vi "newRampTime.vi"(8 "error in (no error)":errorcluster, 11 "RampAction in":refnum<class "RampAction.lvclass">) -> (0 "error out":errorcluster, 3 "RampAction out":refnum<class "RampAction.lvclass">)   [LabVIEW 2009, in "Views.lvlib" / "ScriptEditor.lvlib" / "RampAction.lvclass"]
uses:
  RampAction.lvclass
  RampAction.lvclass/RampAction.ctl
  Tools/Scripting/ScriptingEvent/ScriptEvents/Ramp/RampEvent/RampEvent.lvclass
  ActionPanel.lvclass
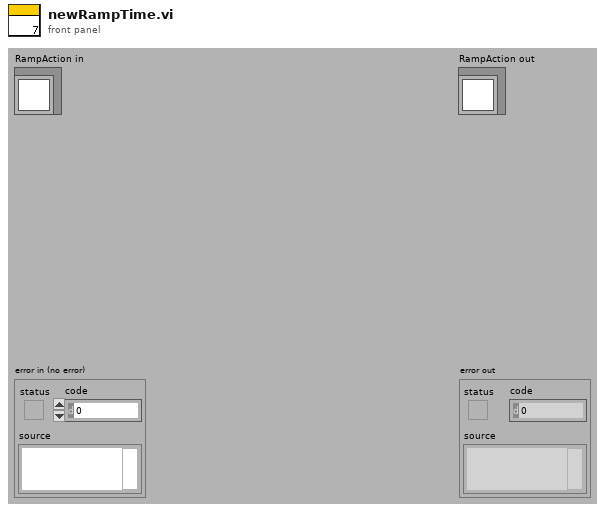
[diagram p1: front panel]
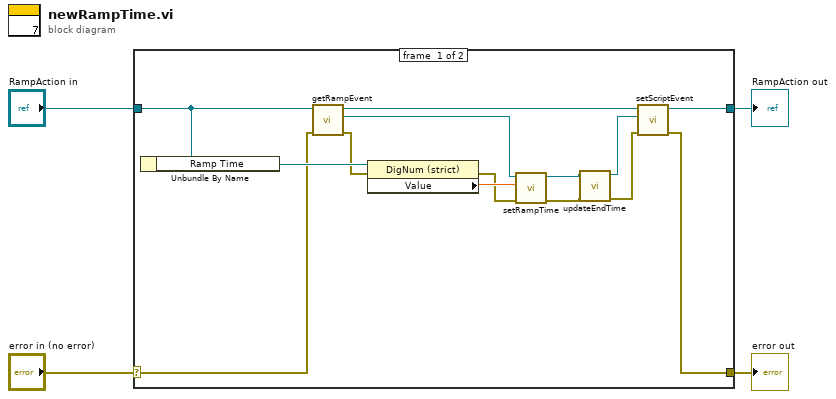
[diagram p0: block diagram]
diagram:
  n1 = case shown="No Error" "error in (no error)" {
    selector: "error in (no error)" -> [w10 w20]
    tunnel: [w9 w20] -> w3
    tunnel: [w11 w19] -> w1
    tunnel: "RampAction in" -> [w17 w19]
    frame #0 {
      n2 = Unbundle By Name(w17) -> ("Ramp Time"=w18:refnum<vi>)
      n3 = call "getRampEvent.vi"("error in (no error)"=w10, "RampAction in"=w17) -> ("error out"=w16:errorcluster, "RampEvent"=w14:refnum<class "RampEvent.lvclass">, "RampAction out"=w12:refnum<class "RampAction.lvclass">)  [unwired: 7 in]
      n4 = property class="DigNum (strict)"(reference=w18, error in=w16) -> (error out=w13:errorcluster, "Value"=w15:dbl)  [unwired: 1 out]
      n5 = call "setRampTime.vi"("error in (no error)"=w13, "rampTime"=w15, "RampEvent.lvclass in"=w14) -> ("error out"=w7:errorcluster, "RampEvent.lvclass out"=w8:refnum<class "RampEvent.lvclass">)  [unwired: 7 in]
      n6 = call-dynamic "updateEndTime.vi"("error in (no error)"=w7, "RampEvent in"=w8) -> ("error out"=w6:errorcluster, "RampEvent out"=w5:refnum<class "RampEvent.lvclass">)  [unwired: 8 in]
      n7 = call "setScriptEvent.vi"("error in (no error)"=w6, "ScriptEvent.lvclass"=w5, "ActionPanel.lvclass in"=w12) -> ("error out"=w9:errorcluster, "ActionPanel.lvclass out"=w11:refnum<class "RampAction.lvclass">)  [unwired: 7 in]
    }
    frame #1 {
    }
  }
  "error out" <- w3
  "RampAction out" <- w1
